vi "VI Tree.vi"   [LabVIEW 2009, in "u-blox 5 Series.lvlib"]
doc: "This is the instrument driver for the u-blox 5 Series. The VI Tree displays all the user-callable VIs of the instrument driver in an organized table."
uses:
  <instrlib>/u-blox 5 Series/u-blox 5 Series.lvlib
panel:
  # "(c) 2009 National Instruments.  ALL RIGHTS RESERVED."
  # "SEE DIAGRAM\nFOR VI TREE."
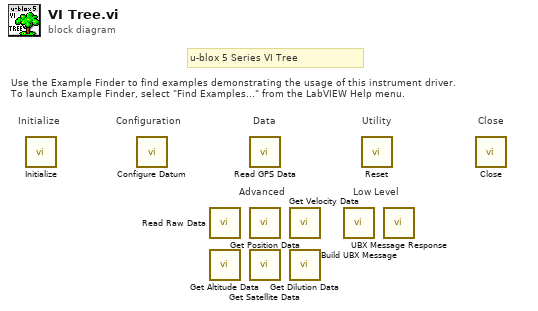
[diagram p0: block diagram]
diagram:
  # "u-blox 5 Series VI Tree"
  # "Use the Example Finder to find examples demonstrating the usage of this instrument driver.\nTo launch Example Finder, select \"Find Examples...\" from the LabVIEW Help menu."
  # "Low Level"
  # "Advanced"
  # "Configuration"
  # "Utility"
  # "Data"
  # "Close"
  # "Initialize"
  n1 = call <instrlib>:"Initialize.vi"() -> ()  [unwired: 10 in, 2 out]
  n2 = call <instrlib>:"Configure Datum.vi"() -> ()  [unwired: 13 in, 3 out]
  n3 = call <instrlib>:"Read Raw Data.vi"() -> ()  [unwired: 8 in, 4 out]
  n4 = call <instrlib>:"Get Altitude Data.vi"() -> ()  [unwired: 8 in, 4 out]
  n5 = call <instrlib>:"Read GPS Data.vi"() -> ()  [unwired: 8 in, 8 out]
  n6 = call <instrlib>:"Get Position Data.vi"() -> ()  [unwired: 8 in, 4 out]
  n7 = call <instrlib>:"Get Satellite Data.vi"() -> ()  [unwired: 8 in, 4 out]
  n8 = call <instrlib>:"Get Velocity Data.vi"() -> ()  [unwired: 8 in, 4 out]
  n9 = call <instrlib>:"Get Dilution Data.vi"() -> ()  [unwired: 8 in, 4 out]
  n10 = call <instrlib>:"Build UBX Message.vi"() -> ()  [unwired: 9 in, 3 out]
  n11 = call <instrlib>:"Reset.vi"() -> ()  [unwired: 9 in, 3 out]
  n12 = call <instrlib>:"UBX Message Response.vi"() -> ()  [unwired: 9 in, 3 out]
  n13 = call <instrlib>:"Close.vi"() -> ()  [unwired: 11 in, 1 out]
